vi "PLC.vi"(8 "error in":errorcluster, 10 "Message Queues":T2, 11 "Notifiers":T3) -> (0 "error out":errorcluster)   [LabVIEW 2015, in "PLC.lvlib"]
uses:
  PLC.lvlib
  Solution/Production Line/support/Message Queue/Message Queue.lvlib
  <vilib>/ErrorRing/Error Ring.xnode
  Model/Model.lvlib
  support/Global names.vi
  <vilib>/Utility/error.llb/Error Cluster From Error Code.vi
  Solution/Production Line/support/Notifiers/Notifiers.ctl
  Solution/Production Line/support/Notifiers/Notifiers.lvlib
  Solution/Production Line/support/Message Queue/Message Cluster.ctl
  Solution/Production Line/support/Message Queue/All Message Queues.ctl
  Type definitions/PLC Data.ctl
panel:
  in  "PLC Data":T1
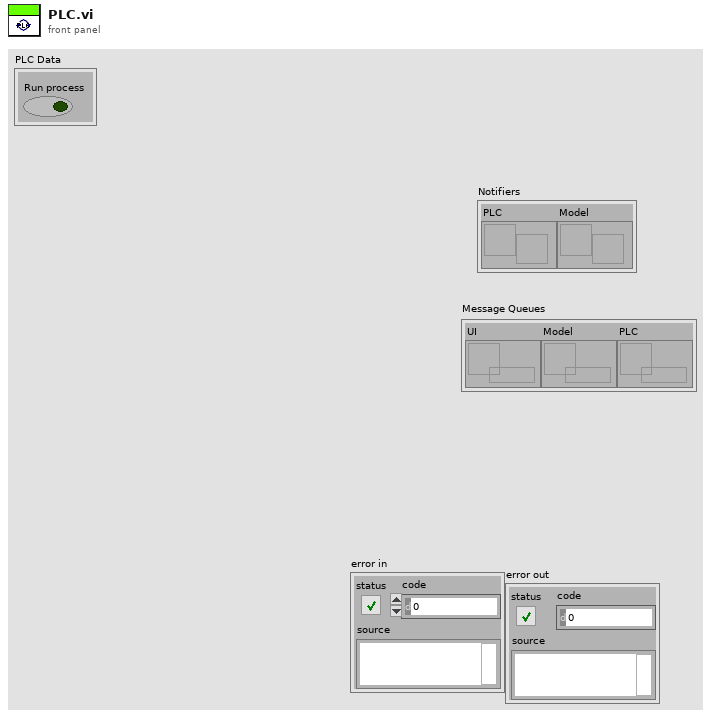
[diagram p1: front panel]
types:
  T1 = typedef "PLC.lvlib/PLC Data.ctl" = cluster{"Run process":bool}
  T2 = typedef "Message Queue.lvlib/All Message Queues.ctl" = cluster{"UI":refnum<queue>, "Model":refnum<queue>, "PLC":refnum<queue>}
  T3 = typedef "Notifiers.lvlib/Notifiers.ctl" = cluster{"PLC":refnum<notifier>, "Model":refnum<notifier>}
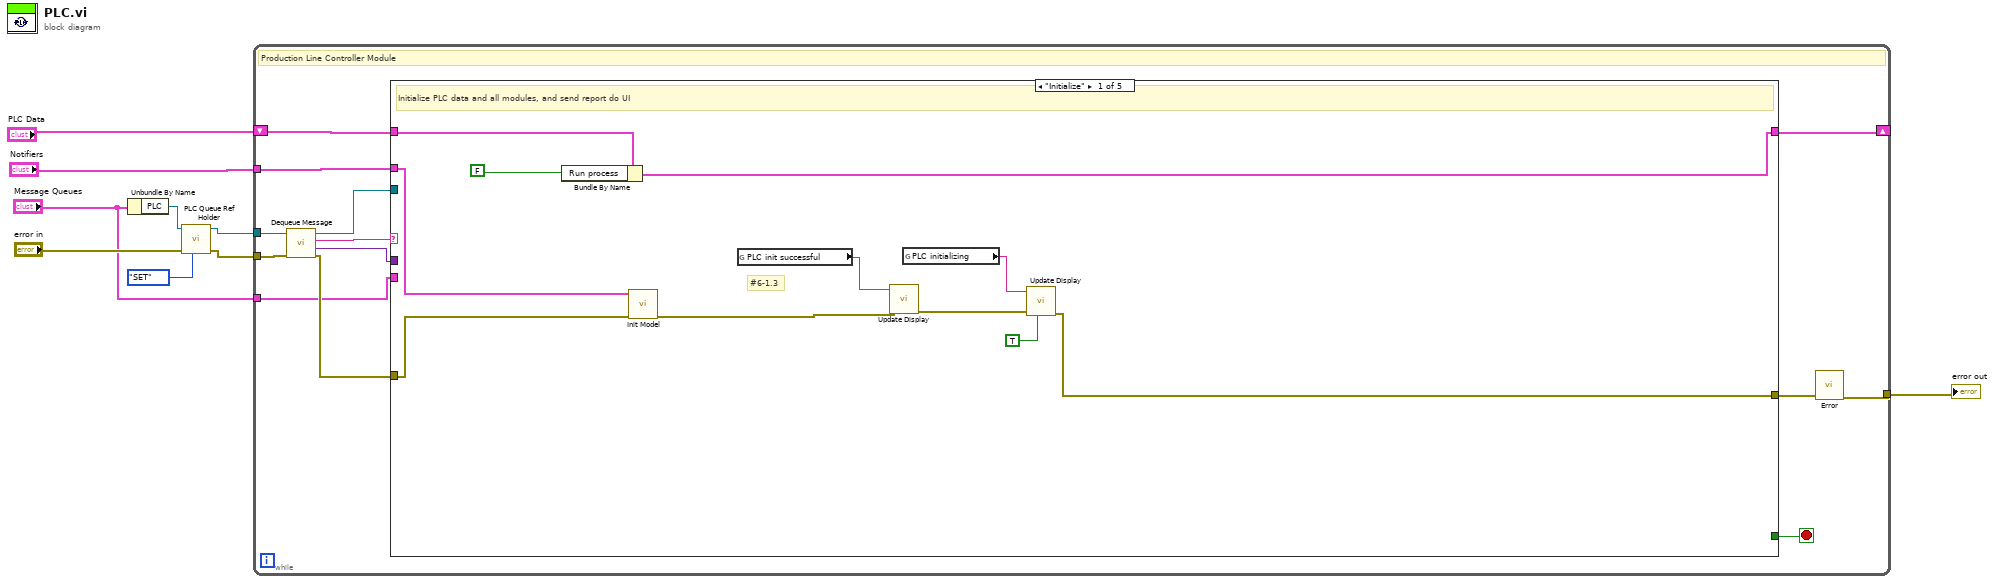
[diagram p0: block diagram]
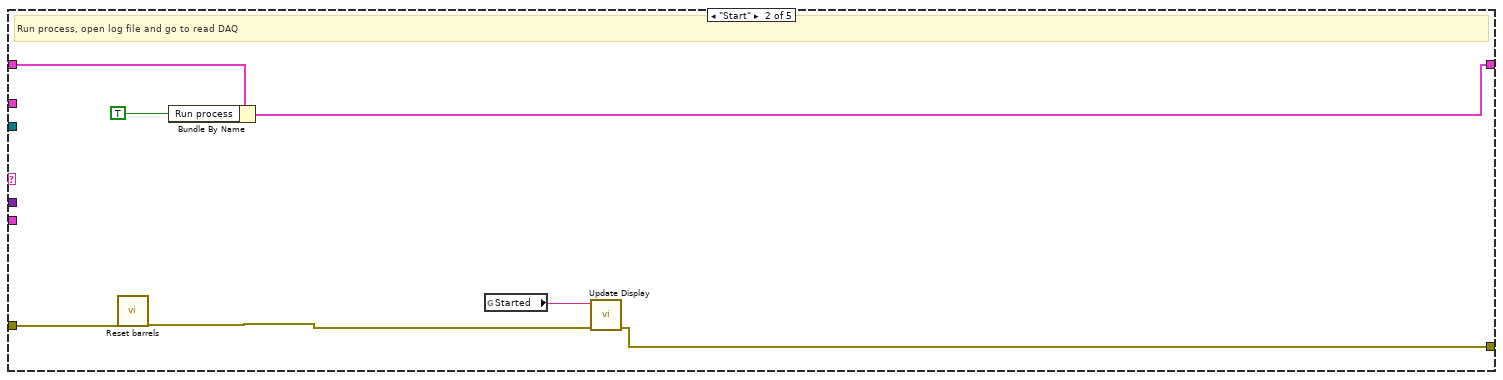
[diagram p2: hidden frame]
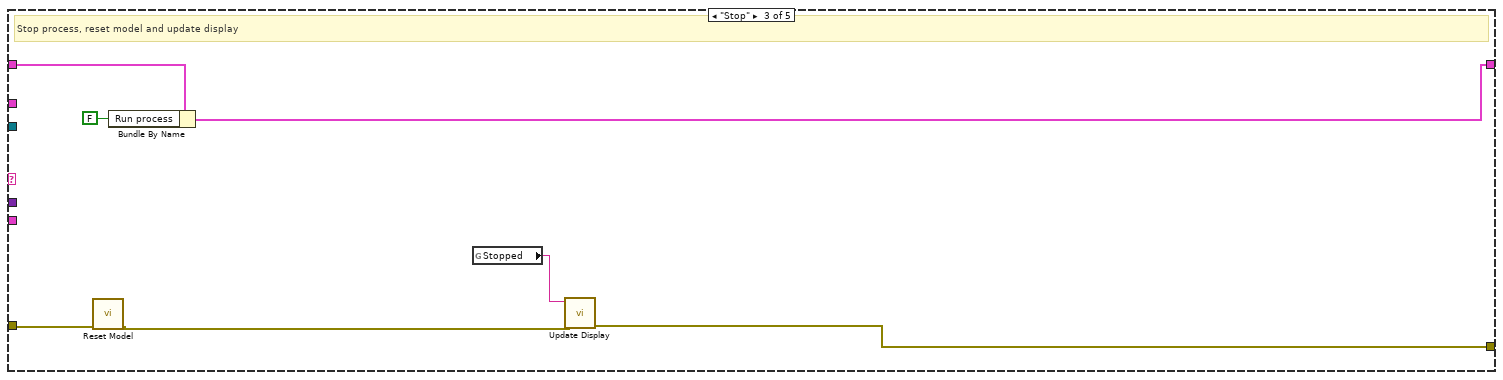
[diagram p3: hidden frame]
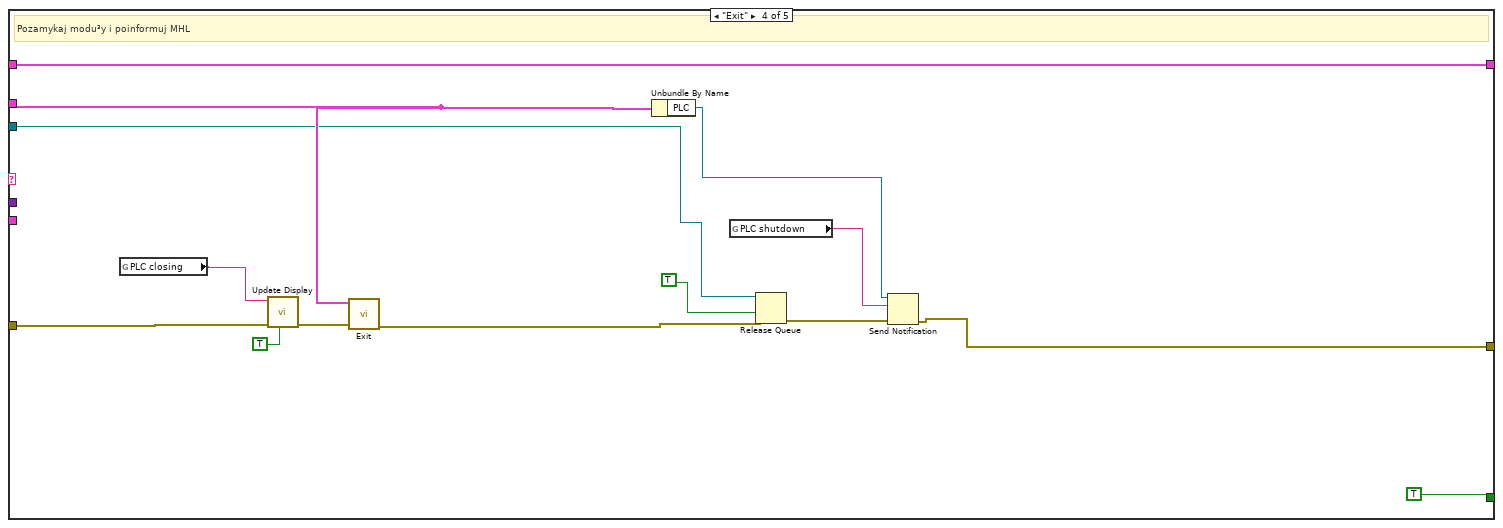
[diagram p4: hidden frame]
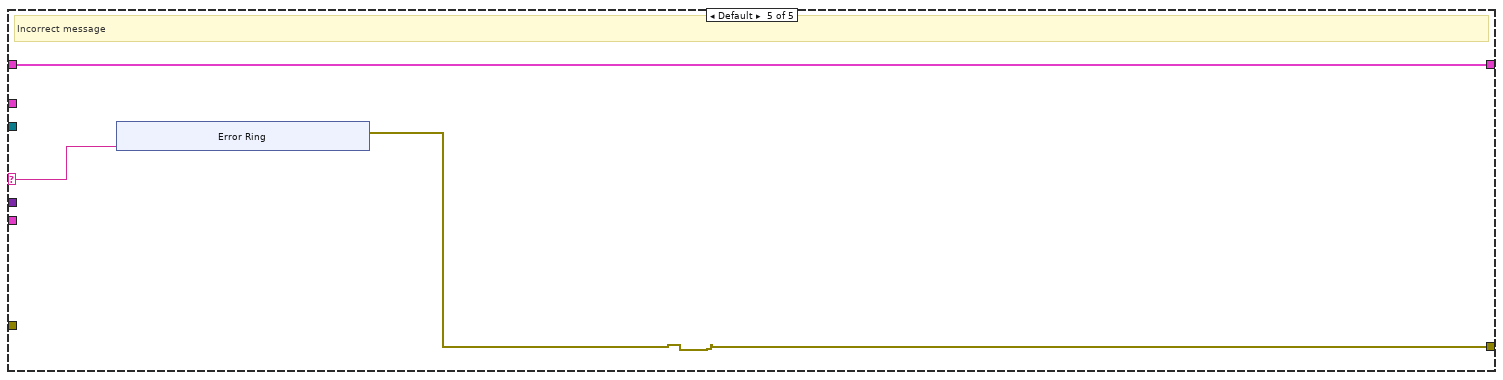
[diagram p5: hidden frame]
diagram:
  n1 = Unbundle By Name("Message Queues") -> ("PLC"=w4:refnum<queue>)
  n2 = call "PLC Queue Ref Holder.vi"("Action"=enum16{"GET", "SET"}."SET", "error in"="error in", "Message Queue In"=w4) -> ("error out"=w5:errorcluster, "Input Message Queue"=w3:refnum<queue>)  [unwired: 7 in]
  n3 = while {
    tunnel: "Notifiers" -> [w22]
    tunnel: w3 -> [w21]
    tunnel: w5 -> [w20]
    tunnel: [w11] -> w9
    tunnel: "Message Queues" -> [w17]
    shift-right: [w15] -> _
    shift-left: "PLC Data" -> [w14]
    stop <- w18 stop-if-true
    # "Production Line Controller Module"
    n4 = call "Dequeue Message.vi"("error in (no error)"=w20, "Message Queue"=w21) -> ("error out"=w19:errorcluster, "Message Data"=w16:variant, "Message"=w10:string, "dup Message Queue"=w13:refnum<queue>)  [unwired: 6 in]
    n5 = case shown="\"Initialize\"" w10 {
      selector: w10 -> [_ _ _ _ w63]
      tunnel: w22 -> [w31 _ _ w59 _]
      tunnel: w19 -> [w30 w35 w43 w49 _]
      tunnel: w13 -> [_ _ _ w51 _]
      tunnel: [_ _ _ TRUE _] -> w18
      tunnel: [w26 w37 w42 w53 w62] -> w12
      tunnel: w17 -> [_ _ _ _ _]
      tunnel: w16 -> [_ _ _ _ _]
      tunnel: w14 -> [w33 w40 w47 w50 w64]
      tunnel: [w32 w39 w45 w50 w64] -> w15
      frame "Initialize" {
        # "#6-1.3"
        # "Initialize PLC data and all modules, and send report do UI"
        n6 = Bundle By Name(cluster=w33, "Run process"=FALSE) -> (w32:T1)
        n7 = call "Init Model.vi"("error in"=w30, "Notifiers in"=w31) -> ("error out"=w28:errorcluster)  [unwired: 8 in, 1 out]
        n8 = global read "Global names.vi" "PLC init successful"() -> (w24:string)
        n9 = call "Update Display.vi"("error in"=w28, "Message string"=w24) -> ("error out"=w27:errorcluster)  [unwired: 9 in]
        n10 = global read "Global names.vi" "PLC initializing"() -> (w23:string)
        n11 = call "Update Display.vi"("Priority Message? (F)"=TRUE, "error in"=w27, "Message string"=w23) -> ("error out"=w26:errorcluster)  [unwired: 8 in]
      }
      frame "Start" {
        # "Run process, open log file and go to read DAQ"
        n12 = call "Reset barrels.vi"("error in"=w35) -> ("error out"=w34:errorcluster)  [unwired: 10 in]
        n13 = Bundle By Name(cluster=w40, "Run process"=TRUE) -> (w39:T1)
        n14 = global read "Global names.vi" "Started"() -> (w36:string)
        n15 = call "Update Display.vi"("error in"=w34, "Message string"=w36) -> ("error out"=w37:errorcluster)  [unwired: 9 in]
      }
      frame "Stop" {
        # "Stop process, reset model and update display"
        n16 = call "Reset Model.vi"("error in"=w43) -> ("error out"=w41:errorcluster)  [unwired: 10 in]
        n17 = Bundle By Name(cluster=w47, "Run process"=FALSE) -> (w45:T1)
        n18 = global read "Global names.vi" "Stopped"() -> (w44:string)
        n19 = call "Update Display.vi"("error in"=w41, "Message string"=w44) -> ("error out"=w42:errorcluster)  [unwired: 9 in]
      }
      frame "Exit" {
        # "Pozamykaj modu³y i poinformuj MHL"
        n20 = global read "Global names.vi" "PLC closing"() -> (w55:string)
        n21 = call "Update Display.vi"("Priority Message? (F)"=TRUE, "error in"=w49, "Message string"=w55) -> ("error out"=w52:errorcluster)  [unwired: 8 in]
        n22 = call "Exit.vi"("error in"=w52, "Notifiers"=w59) -> ("error out"=w48:errorcluster)  [unwired: 9 in]
        n23 = Unbundle By Name(w59) -> ("PLC"=w57:refnum<notifier>)
        n24 = global read "Global names.vi" "PLC shutdown"() -> (w54:string)
        n25 = Release Queue(queue=w51, force destroy? (F)=TRUE, error in (no error)=w48) -> (error out=w60:errorcluster)  [unwired: 2 out]
        n26 = Send Notification(notification=w54, notifier=w57, error in (no error)=w60) -> (error out=w53:errorcluster)  [unwired: 1 out]
      }
      frame Default {
        # "Incorrect message"
        n27 = xnode "Error Ring"("parameter 0"=w63) -> ("error out"=w62:errorcluster)
      }
    }
    n28 = call "Error.vi"("error in"=w12) -> ("error out"=w11:errorcluster)  [unwired: 10 in]
  }
  "error out" <- w9
